vi "GetDiagramOutputs.vi"(6 "error in":errorcluster, 9 "WhileLoop in":refnum<class "WhileLoop.lvclass">) -> (0 "error out":errorcluster, 3 "WhileLoop out":refnum<class "WhileLoop.lvclass">, 4 "output terminals":refnum<class "Terminal.lvclass">[][](array[class]))   [LabVIEW 2014, in "Raspberry Pi Compatible Compiler for LabVIEW.lvlib" / "WhileLoop.lvclass"]
uses:
  WhileLoop.lvclass
  Terminal/Terminal.lvclass
  Loop/Loop.lvclass/Loop.ctl
  Loop/Loop.lvclass
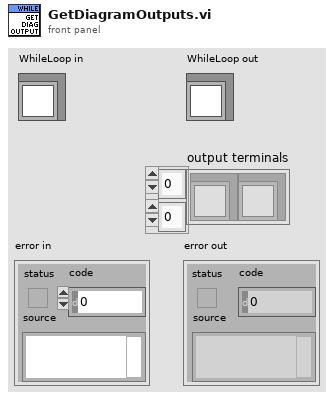
[diagram p1: front panel]
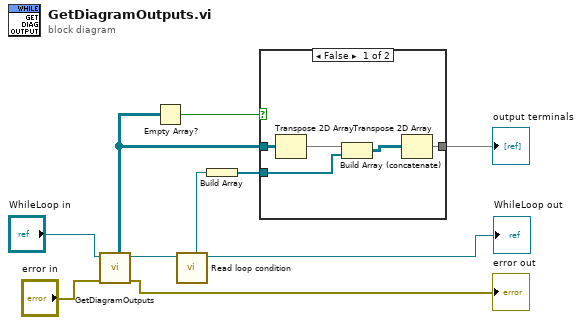
[diagram p0: block diagram]
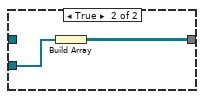
[diagram p2: hidden frame]
diagram:
  n1 = call-parent "GetDiagramOutputs.vi"("error in"="error in", "Loop in"="WhileLoop in") -> ("error out"=→"error out":errorcluster, "Loop out"=w8:refnum<class "WhileLoop.lvclass">, "output terminals"=w2:refnum<class "Terminal.lvclass">[][])  [unwired: 5 in]
  n2 = Empty Array?(array=w2) -> (empty?=w1:bool)
  n3 = call "Read loop condition.vi"("Loop in"=w8) -> ("Loop out"=→"WhileLoop out":refnum<class "WhileLoop.lvclass">, "conditional terminal"=w5:refnum<class "Terminal.lvclass">)  [unwired: 7 in]
  n4 = Build Array(w5) -> (w3:refnum<class "Terminal.lvclass">[])
  n5 = case shown="False" w1 {
    tunnel: [w11 w16] -> w4
    tunnel: w3 -> [w14 w17]
    tunnel: w2 -> [w13 _]
    frame False {
      n6 = Transpose 2D Array(2D array=w13) -> (transposed array=w12:refnum<class "Terminal.lvclass">[][])
      n7 = Build Array (concatenate)(w12, w14) -> (w15:refnum<class "Terminal.lvclass">[][])
      n8 = Transpose 2D Array(2D array=w15) -> (transposed array=w11:refnum<class "Terminal.lvclass">[][])
    }
    frame True {
      n9 = Build Array(w17) -> (w16:refnum<class "Terminal.lvclass">[][])
    }
  }
  "output terminals" <- w4
